vi "Parse_Var_String.vi"(0 "Input":string) -> (1 "Variable name":string="10", 2 "Value":dbl)   [LabVIEW 2012]
panel:
  out "data":string
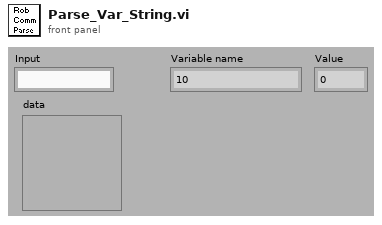
[diagram p1: front panel]
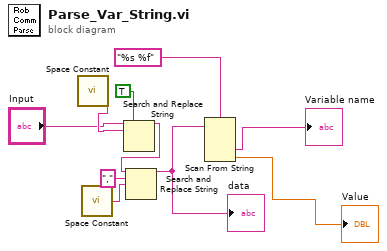
[diagram p0: block diagram]
diagram:
  n1 = call <vilib>:"Space Constant.vi"() -> ("String"=w5:string)
  n2 = call <vilib>:"Space Constant.vi"() -> ("String"=w9:string)
  n3 = Search and Replace String(replace all?=TRUE ("replace all? (F)"), input string="Input", search string=w5) -> (result string=w7:string)  [unwired: 5 in, 3 out]
  n4 = Search and Replace String(input string=w7, search string=",", replace string=w9) -> (result string=w10:string)  [unwired: 5 in, 3 out]
  "data" <- w10
  n5 = Scan From String(format string="%s %f", input string=w10) -> (output 1=→"Variable name":string, output 2=→"Value":dbl)  [unwired: 4 in, 3 out]
